vi "(SubVI)System Command_Board Reset.vi"(8 "error in (no error)":errorcluster caption="에러 입력(에러 없음)") -> (0 "error out":errorcluster caption="에러 출력", 3 "Read Data":u8[](array[numeric]))   [LabVIEW 2020]
uses:
  Serial/Controls/(Ctrl)Serial_Write Read Option.ctl
  09e49390-7250-4416-96e7-00cef826d0ba.vi
  Serial/Instance VIs/(SubVI)Serial_Write.vi
  Serial/Instance VIs/(SubVI)Serial_Write-Read.vi
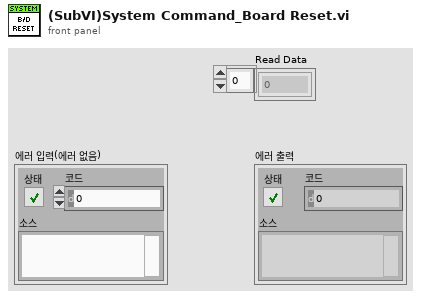
[diagram p1: front panel]
types:
  T1 = typedef "(Ctrl)Serial_Write Read Option.ctl" = cluster{"Echo Request":bool, "Header Verification":bool, "Checksum Verification":bool, "User Code Verifiaction":bool}
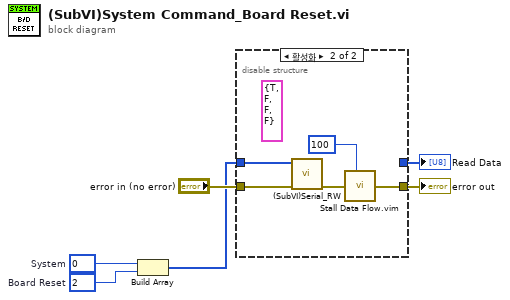
[diagram p0: block diagram]
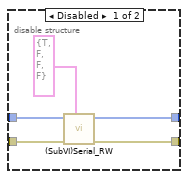
[diagram p2: hidden frame]
diagram:
  w5 = u8 2  # Board Reset
  w6 = u8 0  # System
  n1 = Build Array(w6, w5) -> (w1:u8[])
  n2 = disable-structure shown="활성화" {
    disable-tunnel: [w10 _] -> w4
    disable-tunnel: "error in (no error)" -> [w9 w16]
    disable-tunnel: [w8 w13] -> w2
    disable-tunnel: w1 -> [w7 w14]
    frame Disabled {
      n3 = call-poly "(SubVI)Serial_RW.vi"("Option"=T1 {"Echo Request"=TRUE, "Header Verification"=FALSE, "Checksum Verification"=FALSE, "User Code Verifiaction"=FALSE}, "error in (no error)"=w9, "Data to Write"=w7) -> ("error out"=w8:errorcluster, "Read Data"=w10:u8[])  [unwired: 6 in, 1 out]
    }
    frame Enabled {
      (unwired) T1 {"Echo Request"=TRUE, "Header Verification"=FALSE, "Checksum Verification"=FALSE, "User Code Verifiaction"=FALSE} ("Option")
      n4 = call-poly "(SubVI)Serial_RW.vi"("error in (no error)"=w16, "Data to Write"=w14) -> ("error out"=w15:errorcluster)  [unwired: 9 in]
      n5 = call "Stall Data Flow.vim"("value in"=w15, "milliseconds to wait"=u32 100) -> ("value out"=w13:errorcluster)  [unwired: 1 out]
    }
  }
  "Read Data" <- w4
  "error out" <- w2
